vi "getVariableHeaderLength.vi"(11 "PUBLISH in":refnum<class "PUBLISH.lvclass">) -> (1 "size definitive":bool, 2 "VariableHeader size":u32, 3 "PUBLISH out":refnum<class "PUBLISH.lvclass">)   [LabVIEW 2013, in "MQTT_Control_Packets.lvlib" / "PUBLISH.lvclass"]
uses:
  PUBLISH.lvclass
  ControlPacket/ControlPacket.lvclass/ControlPacket.ctl
  ControlPacket/ControlPacket.lvclass
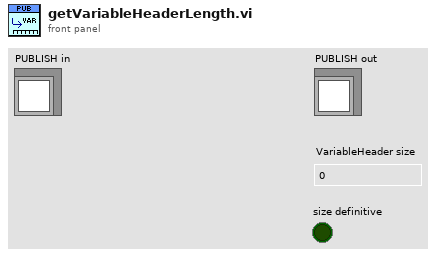
[diagram p1: front panel]
types:
  T1 = typedef "MQTT_Control_Packets.lvlib/ControlPacket.lvclass/QualityOfService -- enum.ctl" = enum16{"0 (At Most Once)", "1 (At Least Once)", "2 (Exactly Once)"}
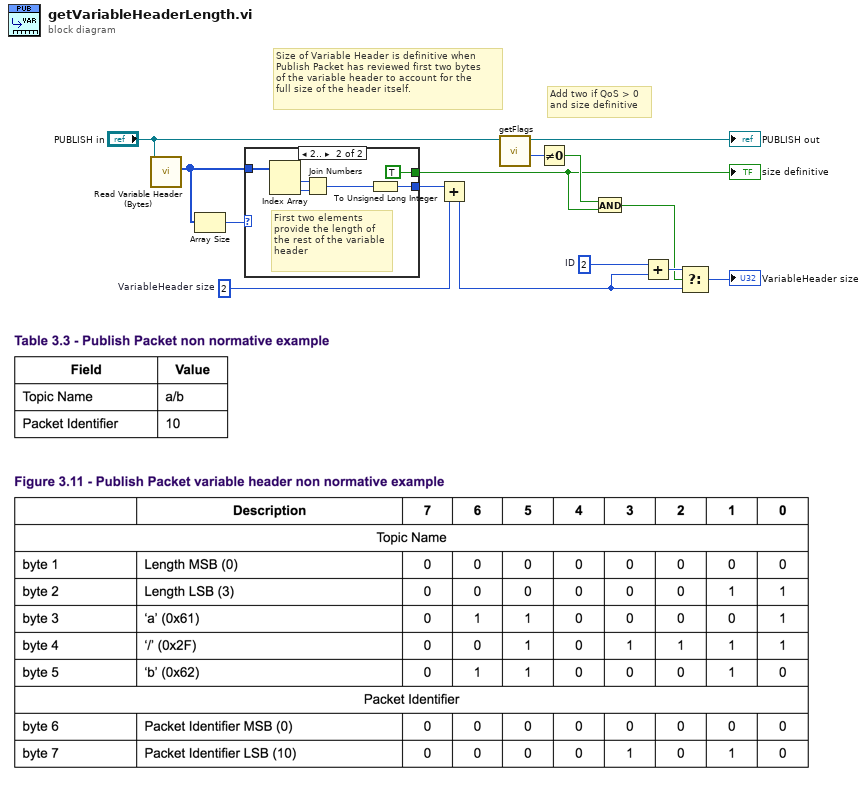
[diagram p0: block diagram]
diagram:
  w4 = u32 2  # ID
  w11 = u32 2  # VariableHeader size
  # "Add two if QoS > 0\nand size definitive"
  # "Size of Variable Header is definitive when\nPublish Packet has reviewed first two bytes\nof the variable header to account for the\nfull size of the header itself."
  n1 = call "Read Variable Header (Bytes).vi"("ControlPacket in"="PUBLISH in") -> ("Variable Header (Bytes)"=w13:u8[])  [unwired: 9 in, 1 out]
  n2 = Array Size(array=w13) -> (size(s)=w14:i32)
  n3 = case shown="2.." w14 {
    tunnel: w13 -> [_ w20]
    tunnel: [_ w17] -> w12
    tunnel: [_ TRUE] -> w1
    frame Default {
    }
    frame 2.. {
      # "First two elements\nprovide the length of\nthe rest of the variable\nheader"
      n4 = Index Array(array=w20) -> (element #1=w18:u8, element #2=w19:u8)  [unwired: 2 in]
      n5 = Join Numbers(hi=w18, lo=w19) -> ((hi.lo)=w15:u16)
      n6 = To Unsigned Long Integer(number=w15) -> (unsigned 32bit integer=w17:u32)
    }
  }
  "size definitive" <- w1
  n7 = Add(x=w12, y=w11) -> (x+y=w3:u32)
  n8 = call-dynamic "getFlags.vi"("PUBLISH in"="PUBLISH in") -> ("QoS"=w7:T1, "PUBLISH out"=→"PUBLISH out":refnum<class "PUBLISH.lvclass">)  [unwired: 7 in, 2 out]
  n9 = Not Equal To 0?(x=w7) -> (x != 0?=w6:bool)
  n10 = And(x=w6, y=w1) -> (x .and. y?=w2:bool)
  n11 = Add(x=w4, y=w3) -> (x+y=w5:u32)
  n12 = Select(t=w5, s=w2, f=w3) -> (s? t:f=→"VariableHeader size":u32)
